vi "Initialize Global Stop.vi"(8 "error in (no error)":errorcluster, 11 "Async in":refnum<class "VS Inline Async API.lvclass">) -> (0 "error out":errorcluster {"code" min=0 max=0}, 3 "Async out":refnum<class "VS Inline Async API.lvclass">)   [LabVIEW 2027, in "VS Inline Async API.lvlib" / "VS Inline Async API.lvclass"]
uses:
  VS Inline Async API.lvclass
  VS Inline Async API.lvclass/VS Inline Async API.ctl
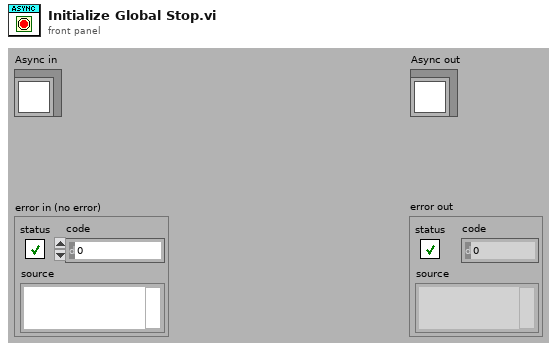
[diagram p1: front panel]
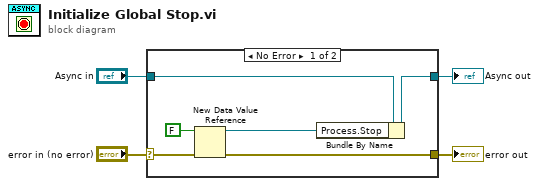
[diagram p0: block diagram]
diagram:
  n1 = case shown="No Error" "error in (no error)" {
    selector: "error in (no error)" -> [w7 w12]
    tunnel: [w6 w12] -> w4
    tunnel: "Async in" -> [w9 w11]
    tunnel: [w8 w11] -> w2
    frame No Error {
      n2 = New Data Value Reference(data value=FALSE, error in=w7) -> (data value reference=w5:refnum<data-value>, error out=w6:errorcluster)
      n3 = Bundle By Name(cluster=w9, "Process.Stop"=w5) -> (w8:refnum<class "VS Inline Async API.lvclass">)
    }
    frame Error {
    }
  }
  "error out" <- w4
  "Async out" <- w2
